vi "POST (Multipart).vi"(6 "timeout":i32=10000, 7 "output file":path, 8 "error in":errorcluster, 9 "Multipart Post data":T1[](array[typedef]), 10 "url":string, 11 "http-method in":refnum<class "REST Client.lvclass">) -> (0 "error out":errorcluster, 2 "response":refnum<class "response.lvclass">, 3 "http-method out":refnum<class "REST Client.lvclass">)   [LabVIEW 2020, in "REST Client.lvlib" / "REST Client.lvclass"]
uses:
  REST Client.lvclass
  response/response.lvclass
  <vilib>/httpClient/MultipartData.ctl
  http-client/http-client.lvclass
  REST Client.lvclass/REST Client.ctl
  <vilib>/httpClient/LabVIEWHTTPClient.lvlib
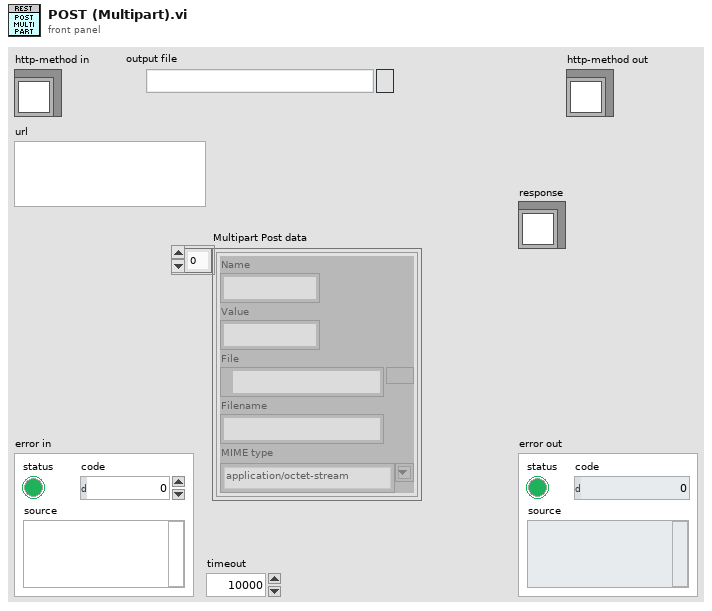
[diagram p1: front panel]
types:
  T1 = typedef "LabVIEWHTTPClient.lvlib/MultipartData.ctl" = cluster{"Name":string, "Value":string, "File":path, "Filename":string, "MIME type":string}
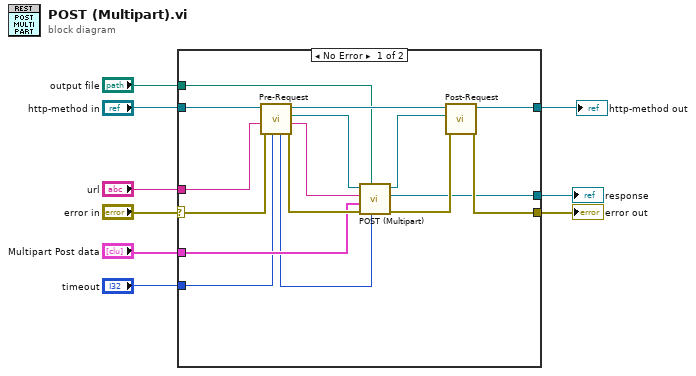
[diagram p0: block diagram]
diagram:
  n1 = case shown="No Error" "error in" {
    selector: "error in" -> [w21 w27]
    tunnel: [w17 w27] -> w4
    tunnel: [w19 w26] -> w3
    tunnel: "http-method in" -> [w20 w26]
    tunnel: "url" -> [w10 _]
    tunnel: "timeout" -> [w12 _]
    tunnel: "Multipart Post data" -> [w18 _]
    tunnel: [w16 _] -> w2
    tunnel: "output file" -> [w15 _]
    frame No Error {
      n2 = call "Pre-Request.vi"("timeout"=w12, "error in (no error)"=w21, "url"=w10, "REST Client in"=w20) -> ("error out"=w23:errorcluster, "Resolved URL"=w24:string, "http-client"=w14:refnum<class "http-client.lvclass">, "REST Client out"=w25:refnum<class "REST Client.lvclass">, "Timeout"=w11:i32)  [unwired: 3 in]
      n3 = call-dynamic "POST (Multipart).vi"("timeout"=w11, "output file"=w15, "error in"=w23, "Multipart Post data"=w18, "url"=w24, "http-method in"=w14) -> ("error out"=w22:errorcluster, "response"=w16:refnum<class "response.lvclass">, "http-method out"=w13:refnum<class "http-client.lvclass">)  [unwired: 3 in]
      n4 = call "Post-Request.vi"("error in (no error)"=w22, "http-method in"=w13, "REST Client in"=w25) -> ("error out"=w17:errorcluster, "REST Client out"=w19:refnum<class "REST Client.lvclass">)  [unwired: 7 in]
    }
    frame Error {
    }
  }
  "error out" <- w4
  "http-method out" <- w3
  "response" <- w2
